vi "ReadFast.vi"(8 "error in (no error)":errorcluster, 10 "Unable to keep up indicator":refnum<vi>, 11 "TDCManager":T1) -> (0 "error out":errorcluster)   [LabVIEW 2016]
uses:
  HPTDC Driver Library Folder/Library files/Typedefs/TDCManagerRefnum.ctl
  HPTDC Driver Library Folder/Library files/Typedefs/TDCManager.ctl
  C:/Users/CRT Controller/CRTC Labview Application/Source/HPTDC Driver Library Folder/Library files/hptdc_net4_3.7.0_x64.dll
  HPTDC Driver Library Folder/Library files/hptdc_net4_3.7.0_x64.dll
  Global Variables/AllowTDCFastRead.vi
  HPTDC Driver Library Folder/HPTDC Driver Library.lvlib
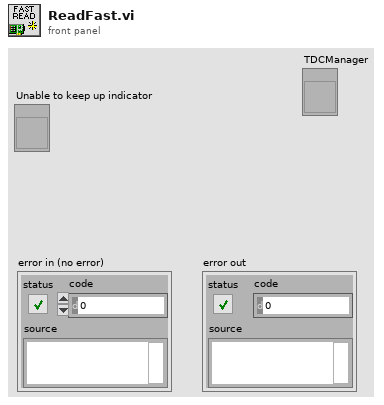
[diagram p1: front panel]
types:
  T1 = typedef "TDCManagerRefnum.ctl" = refnum<vi>
  T2 = enum16{"Reset", "ReadAndReset", "Read", "Add", "Init"}
  T3 = typedef "HPTDC Driver Library.lvlib/TDCManager.ctl" = refnum<k24>
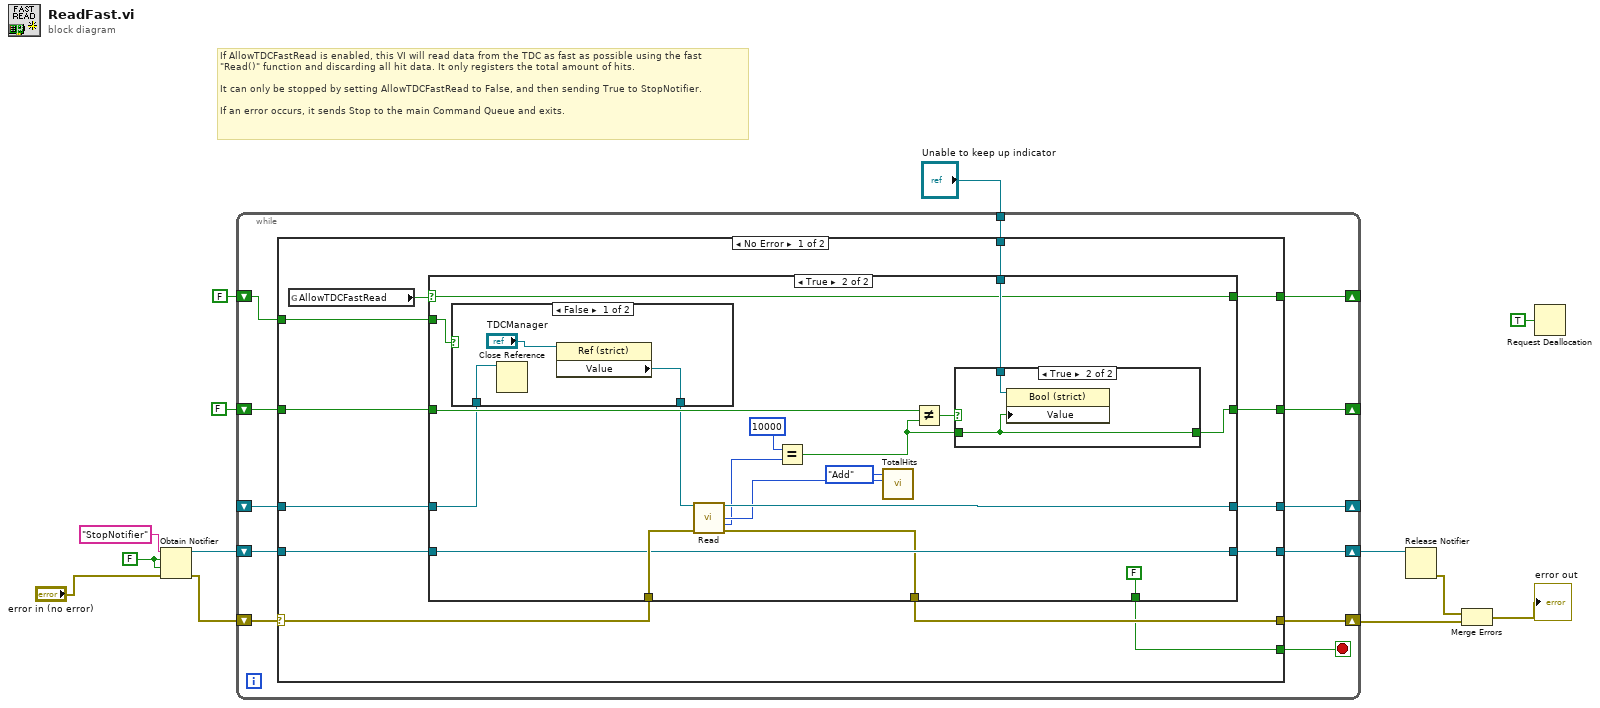
[diagram p0: block diagram]
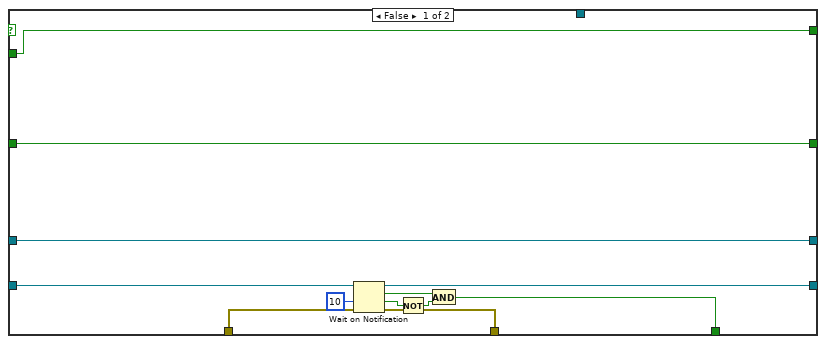
[diagram p2: hidden frame]
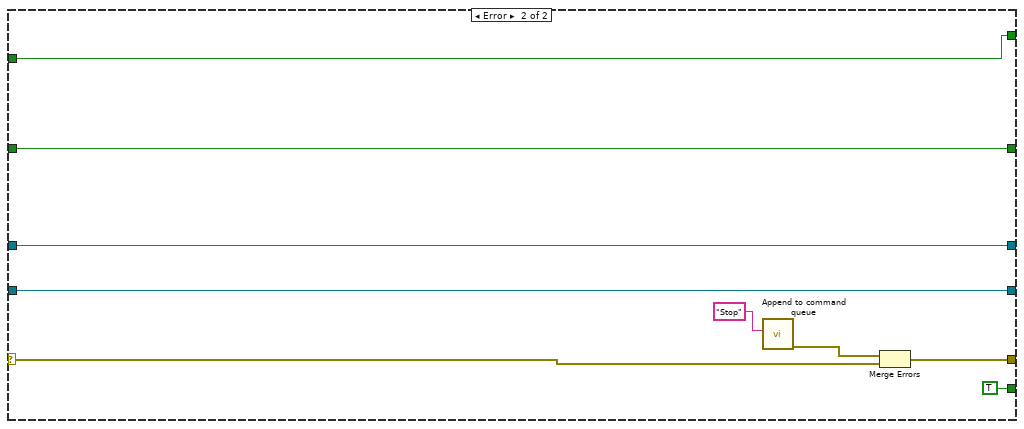
[diagram p5: hidden frame]
diagram:
  w10 = FALSE
  # "If AllowTDCFastRead is enabled, this VI will read data from the TDC as fast as possible using the fast\n\"Read()\" function and discarding all hit data. It only registers the total amount of hits.\n\nIt can only be stopped by setting AllowTDCFastRead to False, and then sending True to StopNotifier.\n\nIf an error occurs, it sends Stop to the main Command Queue and exits."
  n1 = Obtain Notifier(name (unnamed)="StopNotifier", notification data type=w10, create if not found? (T)=w10, error in (no error)="error in (no error)") -> (notifier out=w11:refnum<notifier>, error out=w12:errorcluster)  [unwired: 1 out]
  n2 = while {
    shift-right: [w24] -> w2
    shift-left: w12 -> [w19]
    shift-right: [w23] -> _
    shift-left: _ -> [w25]
    shift-right: [w21] -> w4
    shift-left: w11 -> [w22]
    shift-right: [w18] -> _
    shift-left: FALSE ("timed out?") -> [w17]
    tunnel: "Unable to keep up indicator" -> [w16]
    shift-right: [w15] -> _
    shift-left: FALSE -> [w14]
    stop <- w20 stop-if-true
    n3 = case shown="No Error" w19 {
      selector: w19 -> [w32 w78]
      tunnel: w25 -> [w26 w82]
      tunnel: [w38 w79] -> w24
      tunnel: [w37 w82] -> w23
      tunnel: w22 -> [w35 w83]
      tunnel: [w34 w83] -> w21
      tunnel: [w33 TRUE] -> w20
      tunnel: [w31 w77] -> w18
      tunnel: w17 -> [w30 w77]
      tunnel: w16 -> [w29 _]
      tunnel: [w28 w76] -> w15
      tunnel: w14 -> [w27 w76]
      frame No Error {
        n4 = global read "AllowTDCFastRead.vi" "AllowTDCFastRead"() -> (w36:bool)
        n5 = case shown="True" w36 {
          selector: w36 -> [_ w60]
          tunnel: w26 -> [w50 w58]
          tunnel: w32 -> [w48 w68]
          tunnel: [w47 w57] -> w38
          tunnel: [w50 w67] -> w37
          tunnel: w35 -> [w49 w66]
          tunnel: [w45 w66] -> w34
          tunnel: [w41 FALSE] -> w33
          tunnel: [w40 w62] -> w31
          tunnel: w30 -> [w40 w61]
          tunnel: w29 -> [_ w64]
          tunnel: [w39 w60] -> w28
          tunnel: w27 -> [w39 w59]
          frame False {
            n6 = Wait on Notification(notifier=w49, timeout in ms (-1)=10, error in (no error)=w48) -> (notifier out=w45:refnum<notifier>, notification=w42:bool, timed out?=w44:bool, error out=w47:errorcluster)  [unwired: 1 in]
            n7 = Not(x=w44) -> (.not. x?=w43:bool)
            n8 = And(x=w42, y=w43) -> (x .and. y?=w41:bool)
          }
          frame True {
            n9 = case shown="False" w59 {
              tunnel: w58 -> [w71 w72]
              tunnel: [w69 w72] -> w51
              frame False {
                n10 = Close Reference(reference=w71) -> ()  [unwired: 1 in, 1 out]
                n11 = property on="Property Node" class="Ref (strict)"(reference="TDCManager") -> ("Value"=w69:T3)  [unwired: 1 in, 2 out]
              }
              frame True {
              }
            }
            n12 = call "Read.vi"("TDCManager"=w51, "error in (no error)"=w68) -> ("TDCManager"=w67:T3, "Hits"=w53:i32, "Words read"=w52:i32, "error out"=w57:errorcluster)  [unwired: 9 in, 1 out]
            n13 = Equal?(x=10000, y=w52) -> (x = y?=w55:bool)
            n14 = call "TotalHits.vi"("Number (0)"=w53, "Action"=T2."Add") -> ()  [unwired: 9 in, 1 out]
            n15 = Not Equal?(x=w61, y=w55) -> (x != y?=w63:bool)
            n16 = case shown="True" w63 {
              tunnel: w64 -> [_ w75]
              tunnel: w55 -> [w73 w74]
              tunnel: [w73 w74] -> w62
              frame False {
              }
              frame True {
                n17 = property class="Bool (strict)"(reference=w75, "Value"=w74) -> ()  [unwired: 1 in, 2 out]
              }
            }
          }
        }
      }
      frame Error {
        n18 = call "Append to command queue.vi"("Single command"="Stop") -> ("error out"=w80:errorcluster)  [unwired: 10 in]
        n19 = Merge Errors(w80, w78) -> (w79:errorcluster)
      }
    }
  }
  n20 = Release Notifier(notifier=w4) -> (error out=w3:errorcluster)  [unwired: 2 in, 2 out]
  n21 = Merge Errors(w3, w2) -> (→"error out":errorcluster)
  n22 = Request Deallocation(TRUE ("flag")) -> ()
